vi "sc_CommandSerial.vi"(7 "Query?":bool=TRUE, 8 "error in (no error)":errorcluster, 9 "argument":string, 10 "Scientifica commands":T1=enum."P", 11 "VISA handle":refnum<visa-resource-name>) -> (0 "error out":errorcluster, 2 "Response":string, 3 "Dup. VISA handle":refnum<visa-resource-name>, 5 "TimeoutFlag":bool)   [LabVIEW 2019]
uses:
  controls/scientifica_commands.ctl
panel:
  in  "Array":string[](array[string])
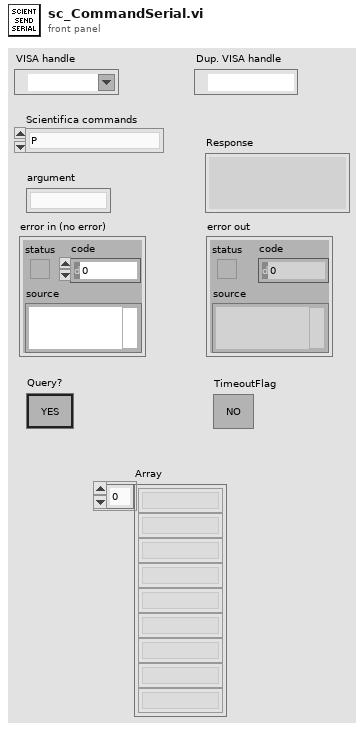
[diagram p1: front panel]
types:
  T1 = typedef "scientifica_commands.ctl" = enum16{"ANGLE", "INSET", "FIRST", "ZERO", "Pz", "P", "absz", "ACC", "TOP", "STOP", "rel", "relz", "abs", "IN", "vj", "APROACH", "OBJS", "OBJU", "OUT", "OBJ", "OBJL", "SET", "OBJD", "STEP", "SETSTEP", "S", "UUX", "UUY", "UUZ"}
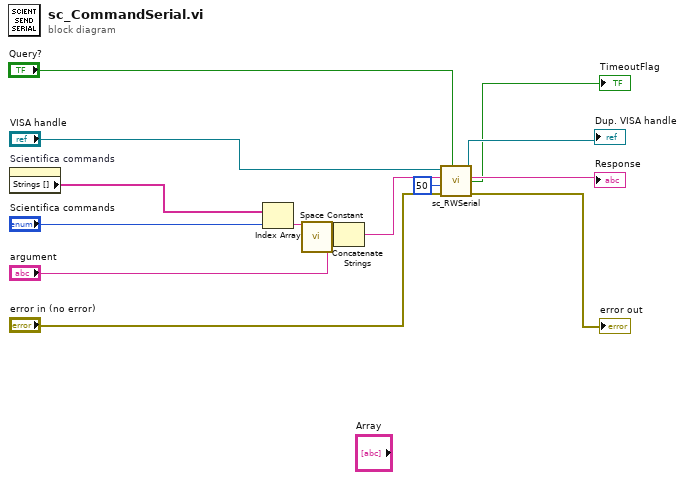
[diagram p0: block diagram]
diagram:
  n1 = property on="Scientifica commands" class="Enum (strict)"() -> ("Strings []"=w8:string[])  [unwired: 2 in, 2 out]
  n2 = Index Array(array=w8, index="Scientifica commands") -> (element=w9:string)
  n3 = call <vilib>:"Space Constant.vi"() -> ("String"=w12:string)
  n4 = Concatenate Strings(w9, w12, "argument") -> (w10:string)
  n5 = call "sc_RWSerial.vi"("Query?"="Query?", "error in (no error)"="error in (no error)", "Delay (ms)"=u32 50, "Command"=w10, "VISA handle"="VISA handle") -> ("error out"=→"error out":errorcluster, "Response"=→"Response":string, "Dup. VISA handle"=→"Dup. VISA handle":refnum<visa-resource-name>, "TimeoutFlag"=→"TimeoutFlag":bool)  [unwired: 1 in]
